vi "15-BuildMap.vi"(11 "Risk Array in":u8[][](array[numeric])) -> (0 "Min Risk Array":i32[][](array[numeric]), 1 "Visited Array":bool[][](array[boolean]), 2 "map":T1(c390), 3 "Risk Array out":u8[][](array[numeric]))   [LabVIEW 2019, in "15.lvlib"]
uses:
  15.lvlib
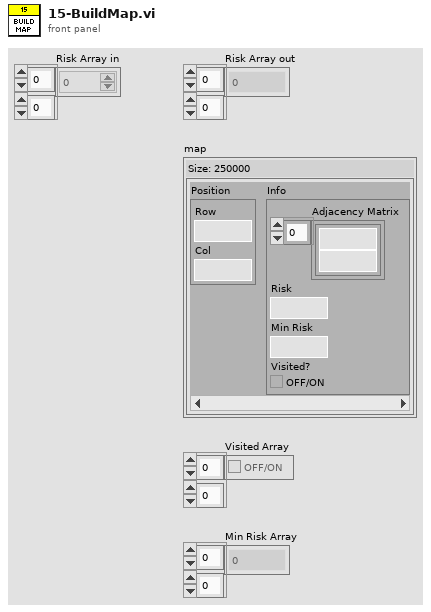
[diagram p1: front panel]
types:
  T1 = map{cluster{"Row":i32, "Col":i32}, cluster{"Adjacency Matrix":cluster{i32, i32}[], "Risk":u8, "Min Risk":i32, "Visited?":bool}}
  T2 = cluster{"Adjacency Matrix":cluster{i32, i32}[], "Risk":u8, "Min Risk":i32, "Visited?":bool}
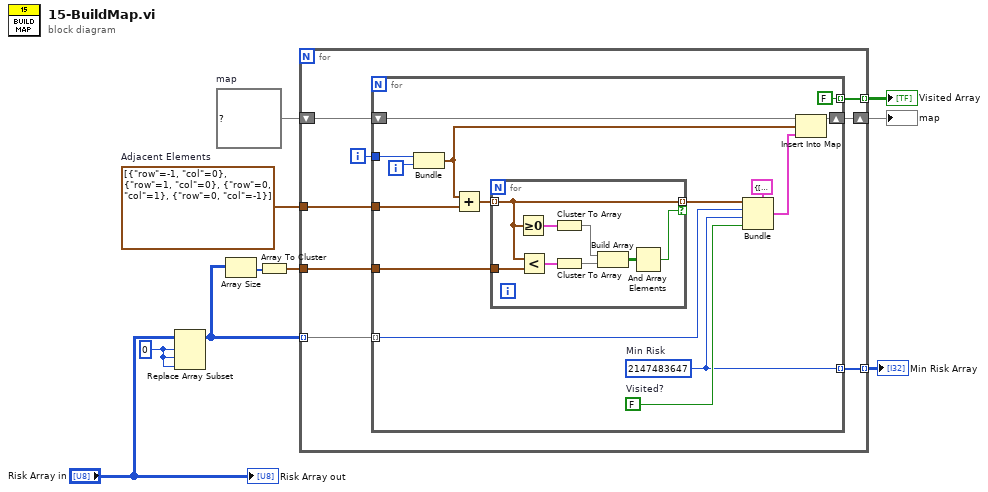
[diagram p0: block diagram]
diagram:
  w3 = 0 ("index")
  w6 = T1 {}  # map
  w2 = cluster{"row":i32, "col":i32}[] [{"row"=-1, "col"=0}, {"row"=1, "col"=0}, {"row"=0, "col"=1}, {"row"=0, "col"=-1}]  # Adjacent Elements
  n1 = Replace Array Subset(array="Risk Array in", new element=w3, index (row)=w3, index (col)=w3) -> (w10:u8[][])
  n2 = Array Size(array=w10) -> (size(s)=w4:i32[])
  n3 = Array To Cluster(array=w4) -> (cluster=w5:cluster{"[0]":i32, "[1]":i32})
  n4 = for {
    tunnel: w10 -> [w16] mode=indexing
    tunnel: w2 -> [w17]
    shift-right: [w15] -> w8
    shift-left: w6 -> [w14]
    tunnel: w5 -> [w13]
    tunnel: [w12] -> w7 mode=indexing
    tunnel: [w11] -> w1 mode=indexing
    i -> [w18]
    n5 = for {
      tunnel: w18 -> [w30]
      tunnel: w17 -> [w31]
      tunnel: w16 -> [w21] mode=indexing
      shift-right: [w32] -> w15
      shift-left: w14 -> [w33]
      tunnel: w13 -> [w26]
      tunnel: [FALSE] -> w12 mode=indexing
      tunnel: [w19] -> w11 mode=indexing
      i -> [w29]
      w19 = 2147483647  # Min Risk
      w24 = FALSE  # Visited?
      n6 = Bundle(w30, w29) -> (w23:cluster{i32, i32})  [unwired: 1 in]
      n7 = Add(x=w23, y=w31) -> (x+y=w27:cluster{i32, i32}[])
      n8 = for {
        tunnel: w27 -> [w35] mode=indexing
        tunnel: w26 -> [w41]
        tunnel: [w35] -> w25 mode=indexing if=w34
        n9 = Greater Or Equal To 0?(x=w35) -> (x >= 0?=w40:cluster{bool, bool})
        n10 = Less?(x=w35, y=w41) -> (x < y?=w39:cluster{bool, bool})
        n11 = Cluster To Array(cluster=w40) -> (array=w38:bool[])
        n12 = Cluster To Array(cluster=w39) -> (array=w37:bool[])
        n13 = Build Array(w38, w37) -> (w36:bool[][])
        n14 = And Array Elements(Boolean array=w36) -> (logical AND=w34:bool)
      }
      n15 = Bundle(cluster=T2 {"Adjacency Matrix"=[], "Risk"=0, "Min Risk"=0, "Visited?"=FALSE} ("Info"), "Adjacency Matrix"=w25, "Risk"=w21, "Min Risk"=w19, "Visited?"=w24) -> (w28:T2)
      n16 = Insert Into Map(map in=w33, key=w23, value=w28) -> (map out=w32:T1)  [unwired: 2 out]
    }
  }
  "map" <- w8
  "Visited Array" <- w7
  "Min Risk Array" <- w1
  "Risk Array out" <- "Risk Array in"
